vi "LCfiletrans1(SubVI).vi"(8 "error in (no error)":errorcluster, 9 "Source Filename":string, 10 "file path (use dialog)":path, 11 "VISA Refnum in":refnum<visa-resource-name>) -> (0 "error out":errorcluster, 2 "File data":string, 3 "VISA Refnum out":refnum<visa-resource-name>)   [LabVIEW 2018]
uses:
  <instrlib>/LeCroy Wave Series/LeCroy Wave Series.lvlib
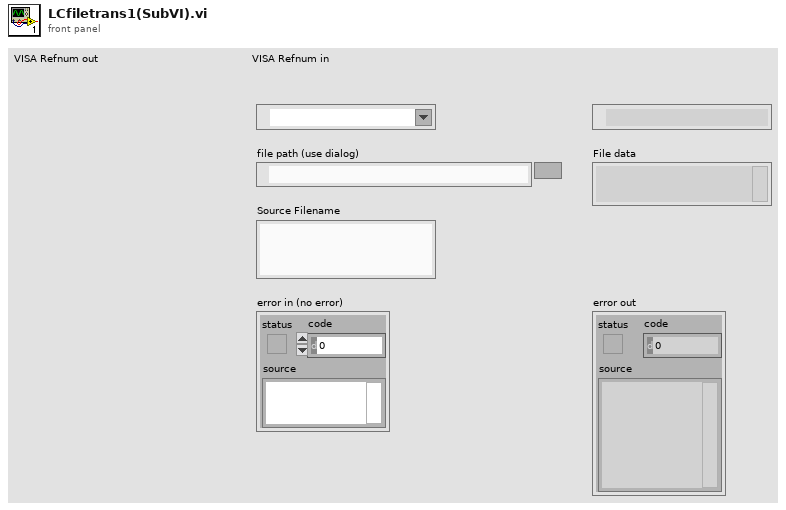
[diagram p1: front panel]
types:
  T1 = enum16{"open", "replace", "create", "open or create", "replace or create", "replace or create with confirmation"}
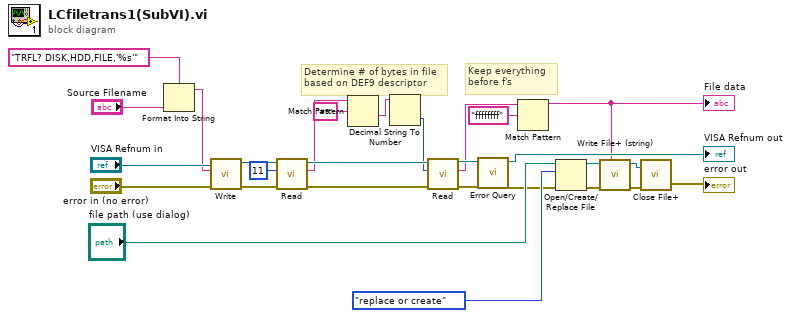
[diagram p0: block diagram]
diagram:
  # "Keep everything \nbefore f's"
  # "Determine # of bytes in file\nbased on DEF9 descriptor"
  n1 = Format Into String(format string="TRFL? DISK,HDD,FILE,'%s'" ("initial string"), "Source Filename") -> (resulting string=w22:string)  [unwired: 2 in, 1 out]
  n2 = call <instrlib>:"Write.vi"("error in (no error)"="error in (no error)", "Write Buffer"=w22, "VISA resource name"="VISA Refnum in") -> ("error out"=w18:errorcluster, "VISA resource name out"=w21:refnum<visa-resource-name>)  [unwired: 7 in]
  n3 = call <instrlib>:"Read.vi"("error in (no error)"=w18, "Byte Count"=u32 11, "VISA resource name"=w21) -> ("error out"=w17:errorcluster, "Read Buffer"=w15:string, "VISA resource name out"=w20:refnum<visa-resource-name>)  [unwired: 5 in, 1 out]
  n4 = Match Pattern(string=w15, regular expression="#9") -> (after substring=w13:string)  [unwired: 1 in, 3 out]
  n5 = Decimal String To Number(string=w13) -> (number=w12:i32)  [unwired: 2 in, 1 out]
  n6 = call <instrlib>:"Read.vi"("error in (no error)"=w17, "Byte Count"=w12, "VISA resource name"=w20) -> ("error out"=w7:errorcluster, "Read Buffer"=w10:string, "VISA resource name out"=w19:refnum<visa-resource-name>)  [unwired: 5 in, 1 out]
  n7 = call <instrlib>:"Error Query.vi"("error in (no error)"=w7, "VISA resource name"=w19) -> ("error out"=w6:errorcluster, "VISA resource name out"=→"VISA Refnum out":refnum<visa-resource-name>)  [unwired: 6 in, 2 out]
  n8 = Match Pattern(string=w10, regular expression="ffffffff") -> (before substring=w1:string)  [unwired: 1 in, 3 out]
  "File data" <- w1
  n9 = Open/Create/Replace File(file path (use dialog)="file path (use dialog)", error in=w6, operation (0:open)=T1."replace or create") -> (refnum out=w5:refnum<file>, error out=w9:errorcluster)  [unwired: 3 in, 1 out]
  n10 = call <vilib>:"Write File+ (string).vi"("string"=w1, "error in (no error)"=w9, "refnum"=w5) -> ("error out"=w8:errorcluster, "dup refnum"=w4:refnum<file>)  [unwired: 4 in, 1 out]
  n11 = call <vilib>:"Close File+.vi"("error in (no error)"=w8, "refnum"=w4) -> ("error out"=→"error out":errorcluster)  [unwired: 3 in, 2 out]
